vi "Reading buffer basetimestamp.vi"(8 "错误输入":errorcluster, 10 "缓冲区名称":string(combo), 11 "VISA资源名称":refnum<visa-resource-name>) -> (0 "错误输出":errorcluster, 2 "时间标识":timestamp, 3 "VISA资源名称输出":refnum<visa-resource-name>)   [LabVIEW 2019]
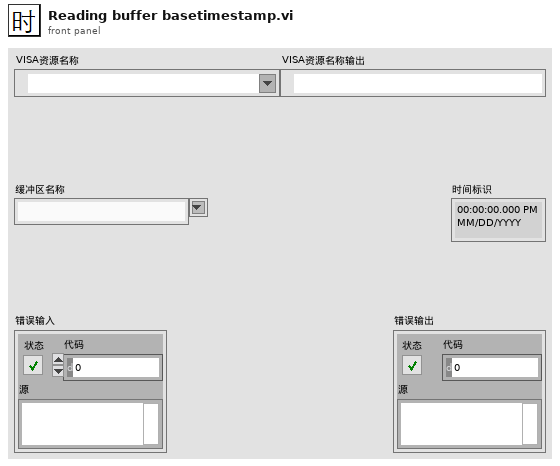
[diagram p1: front panel]
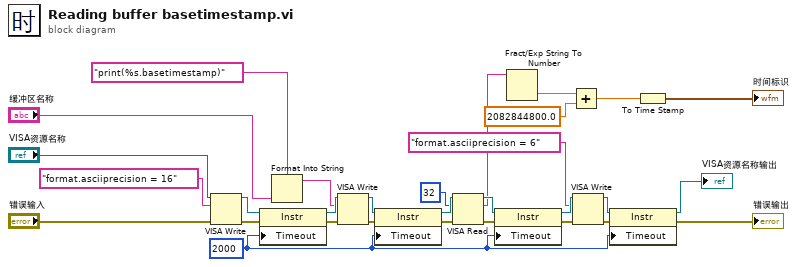
[diagram p0: block diagram]
diagram:
  w6 = u32 2000 ("General Settings:Timeout Value")
  n1 = VISA Write(VISA resource name="VISA资源名称", write buffer="format.asciiprecision = 16" ("格式字符串"), error in (no error)="错误输入") -> (VISA resource name out=w30:refnum<visa-resource-name>, error out=w29:errorcluster)  [unwired: 1 out]
  n2 = property class="Instr"(reference=w30, error in=w29, "Timeout"=w6) -> (reference out=w19:refnum<visa-resource-name>, error out=w18:errorcluster)
  n3 = Format Into String(format string="print(%s.basetimestamp)" ("格式字符串"), "缓冲区名称") -> (resulting string=w11:string)  [unwired: 2 in, 1 out]
  n4 = VISA Write(VISA resource name=w19, write buffer=w11, error in (no error)=w18) -> (VISA resource name out=w28:refnum<visa-resource-name>, error out=w27:errorcluster)  [unwired: 1 out]
  n5 = property class="Instr"(reference=w28, error in=w27, "Timeout"=w6) -> (reference out=w25:refnum<visa-resource-name>, error out=w26:errorcluster)
  n6 = VISA Read(VISA resource name=w25, byte count=u32 32 ("字节总数"), error in (no error)=w26) -> (VISA resource name out=w24:refnum<visa-resource-name>, read buffer=w14:string, error out=w23:errorcluster)  [unwired: 1 out]
  n7 = property class="Instr"(reference=w24, error in=w23, "Timeout"=w6) -> (reference out=w4:refnum<visa-resource-name>, error out=w5:errorcluster)
  n8 = Fract/Exp String To Number(string=w14) -> (number=w12:dbl)  [unwired: 3 in, 1 out]
  n9 = Add(x=w12, y=2082844800.0 ("x-y")) -> (x+y=w10:dbl)
  n10 = VISA Write(VISA resource name=w4, write buffer="format.asciiprecision = 6" ("格式字符串"), error in (no error)=w5) -> (VISA resource name out=w8:refnum<visa-resource-name>, error out=w7:errorcluster)  [unwired: 1 out]
  n11 = property class="Instr"(reference=w8, error in=w7, "Timeout"=w6) -> (reference out=→"VISA资源名称输出":refnum<visa-resource-name>, error out=→"错误输出":errorcluster)
  n12 = To Time Stamp(1:w10) -> (0:→"时间标识":timestamp)
